vi "set_basic_auth.vi"(8 "error in":errorcluster, 9 "password":string, 10 "username":string, 11 "obj in":refnum<class "RequestBuilder.lvclass">) -> (0 "error out":errorcluster, 2 "success":bool, 3 "obj out":refnum<class "RequestBuilder.lvclass">)   [LabVIEW 2020, in "reqwest.lvlib" / "RequestBuilder.lvclass"]
uses:
  RequestBuilder.lvclass
  RequestBuilder.lvclass/RequestBuilder.ctl
  lv_reqwest_64.dll
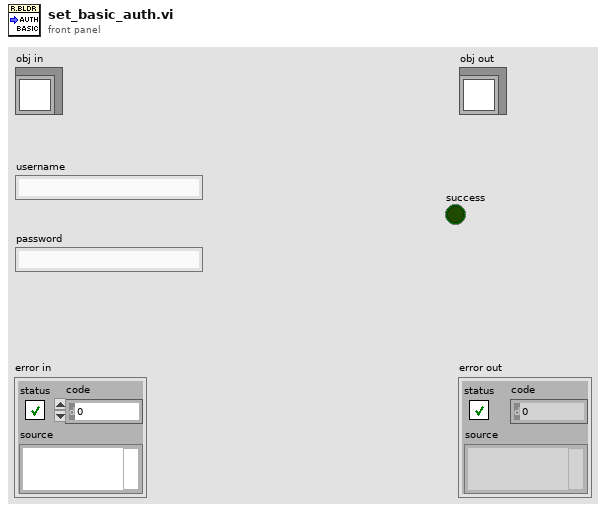
[diagram p1: front panel]
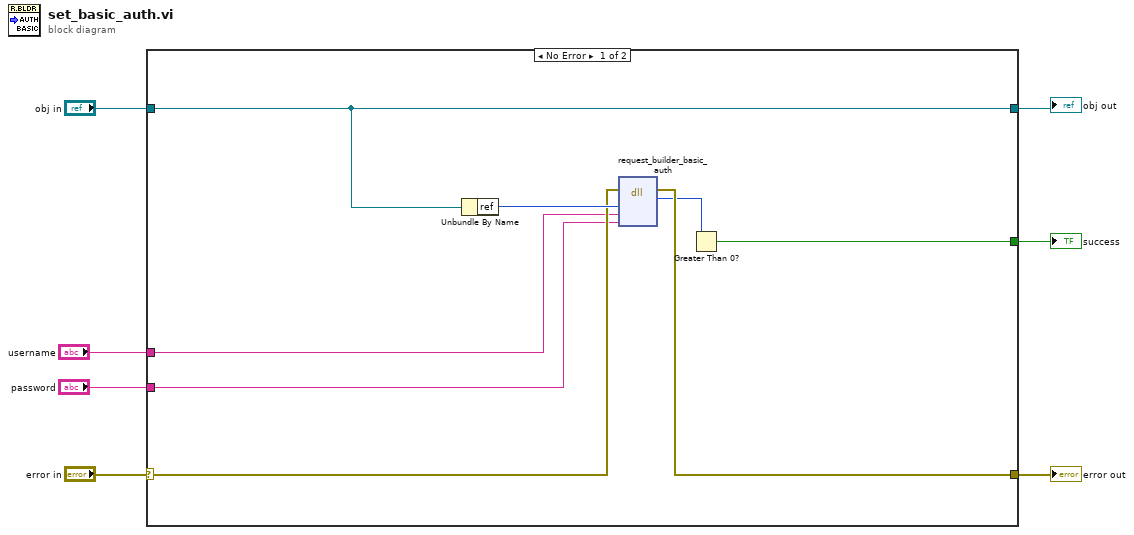
[diagram p0: block diagram]
diagram:
  n1 = case shown="No Error" "error in" {
    selector: "error in" -> [w12 w16]
    tunnel: "obj in" -> [w13 w17]
    tunnel: [w15 w16] -> w4
    tunnel: [w13 w17] -> w5
    tunnel: "username" -> [w9 _]
    tunnel: [w10 _] -> w2
    tunnel: "password" -> [w8 _]
    frame No Error {
      n2 = Unbundle By Name(w13) -> ("ref"=w14:u64)
      n3 = dll-call lib="C:/Projects/vipm-desktop/source/submodules/reqwest-rs-labview/lv_src/lv_reqwest_*.*" fn="request_builder_basic_auth"(error in=w12, "request_builder_ref"=w14, "username"=w9, "password"=w8) -> (error out=w15:errorcluster, "success"=w11:u8)  [unwired: 5 in, 1 out]
      n4 = Greater Than 0?(x=w11) -> (x > 0?=w10:bool)
    }
    frame Error {
    }
  }
  "error out" <- w4
  "obj out" <- w5
  "success" <- w2
